vi "Convert Functional String to Pretty String.vi"(4 "Functional Name":string) -> (1 "Pretty Name":string)   [LabVIEW 2021, in "Strings.lvlib"]
doc: "Replaces underscore by spaces and double underscores by alternating parentheses.\n\nUse this function to convert a file or function name to a more user-friendly display name."
uses:
  Strings.lvlib
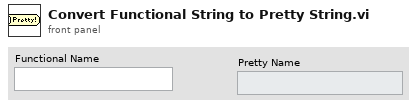
[diagram p1: front panel]
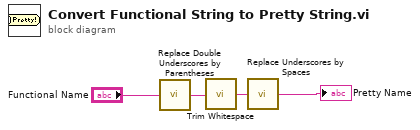
[diagram p0: block diagram]
diagram:
  n1 = call "Replace Double Underscores by Parentheses.vi"("String in"="Functional Name") -> ("String out"=w3:string)  [unwired: 8 in]
  n2 = call <vilib>:"Trim Whitespace.vi"("string"=w3) -> ("trimmed string"=w2:string)  [unwired: 1 in]
  n3 = call "Replace Underscores by Spaces.vi"("String in"=w2) -> ("String out"=→"Pretty Name":string)  [unwired: 8 in]
